vi "Read Sequential Addresses.vi"(7 "Target IC (1-8)":u8, 8 "error in (no error)":errorcluster, 9 "Addresses to Read":u16 format="%0.0f", 10 "Starting Address":u16 format="%04x", 11 "FPGA Interface in":refnum<class "FPGA Interface.lvclass">) -> (0 "error out":errorcluster, 2 "Data":u16[](array[numeric]) format="%04x")   [LabVIEW 2020, in "BCI-1553 API.lvlib" / "FPGA Interface.lvlib" / "FPGA Interface.lvclass"]
doc: "Reads a series of consecutive addresses from a component in the 1553 Session. Sequential addressing cannot be used on addresses from 0x0400 to 0x0800. This command blocks until it receives data back from the specified component."
uses:
  FPGA Interface.lvclass
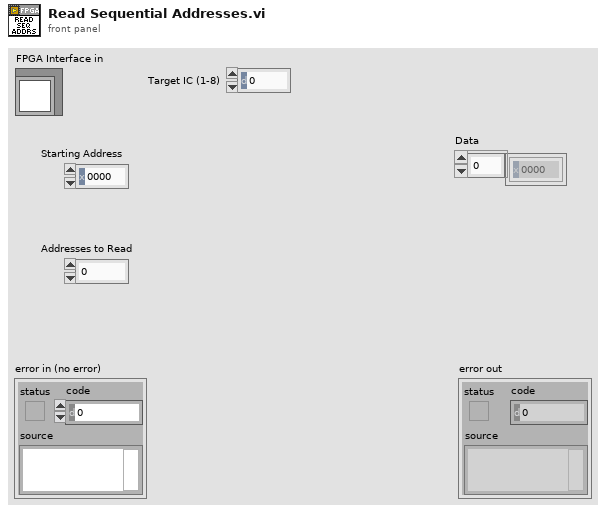
[diagram p1: front panel]
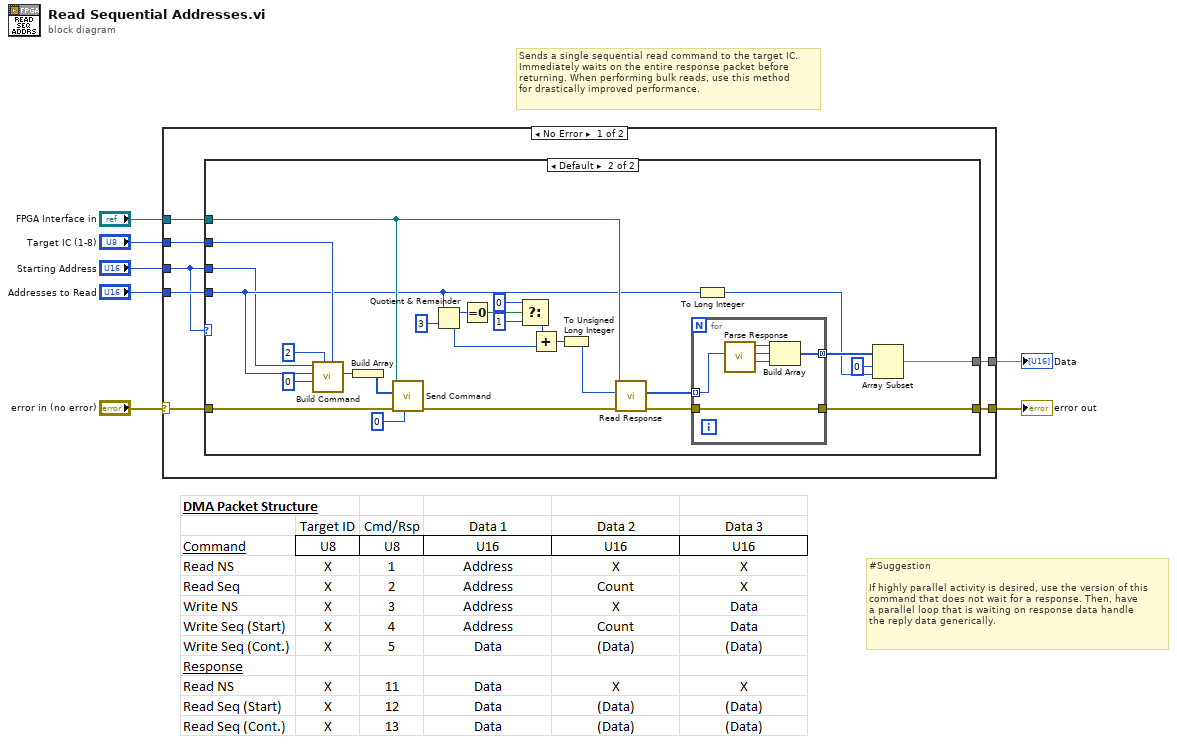
[diagram p0: block diagram]
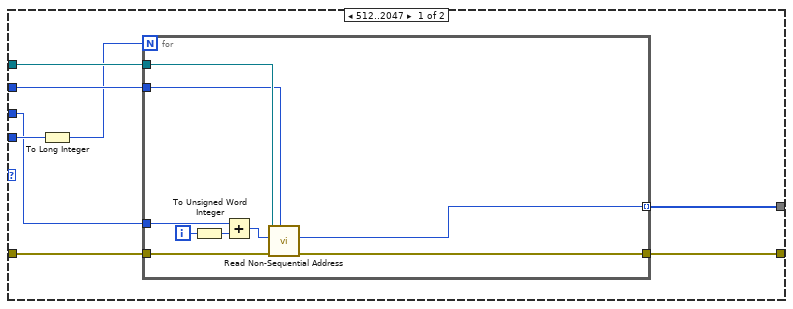
[diagram p2: hidden frame]
diagram:
  # "Sends a single sequential read command to the target IC.\nImmediately waits on the entire response packet before\nreturning. When performing bulk reads, use this method\nfor drastically improved performance."
  # "#Suggestion\n\nIf highly parallel activity is desired, use the version of this\ncommand that does not wait for a response. Then, have\na parallel loop that is waiting on response data handle\nthe reply data generically."
  n1 = case shown="No Error" "error in (no error)" {
    selector: "error in (no error)" -> [w14 w65]
    tunnel: [w11 w65] -> w6
    tunnel: "FPGA Interface in" -> [w12 _]
    tunnel: "Target IC (1-8)" -> [w13 _]
    tunnel: "Starting Address" -> [w8 _]
    tunnel: "Addresses to Read" -> [w9 _]
    tunnel: [w10 _] -> w1
    frame No Error {
      n2 = case shown="Default" w8 {
        tunnel: w14 -> [w17 w54]
        tunnel: w13 -> [w21 w53]
        tunnel: w12 -> [w22 w52]
        tunnel: [w16 w49] -> w11
        tunnel: [w15 w44] -> w10
        tunnel: w9 -> [w20 w43]
        tunnel: w8 -> [w18 w33]
        frame 512..2047 {
          n3 = To Long Integer(number=w20) -> (32bit integer=w19:i32)
          n4 = for {
            N: w19 -> [_]
            tunnel: w22 -> [w31]
            tunnel: w21 -> [w30]
            tunnel: w18 -> [w27]
            tunnel: w17 -> [w25]
            tunnel: [w24] -> w16
            tunnel: [w23] -> w15 mode=indexing
            i -> [w28]
            n5 = To Unsigned Word Integer(number=w28) -> (unsigned 16bit integer=w29:u16)
            n6 = Add(x=w27, y=w29) -> (x+y=w26:u16)
            n7 = call-dynamic "Read Non-Sequential Address.vi"("Target IC (1-8)"=w30, "error in (no error)"=w25, "Address"=w26, "FPGA Interface in"=w31) -> ("error out"=w24:errorcluster, "Data"=w23:u16)  [unwired: 6 in]
          }
        }
        frame Default {
          n8 = call "Build Command.vi"("Target"=w53, "CMD ID"=u8 2, "Data 3"=u16 0, "Data 2"=w43, "Data 1"=w33) -> ("Command"=w58:u64)  [unwired: 5 in, 1 out]
          n9 = Build Array(w58) -> (w57:u64[])
          n10 = call "Send Command.vi"("Timeout (ms)"=0, "error in (no error)"=w54, "Data"=w57, "FPGA Interface in"=w52) -> ("error out"=w56:errorcluster)  [unwired: 7 in]
          n11 = Quotient & Remainder(x=w43, y=u16 3) -> (x-y*floor(x/y)=w38:u16, floor(x/y)=w40:u16)
          n12 = Equal To 0?(x=w38) -> (x = 0?=w37:bool)
          n13 = Select(t=u16 0 ("y"), s=w37, f=u16 1 ("y")) -> (s? t:f=w36:u16)
          n14 = Add(x=w36, y=w40) -> (x+y=w39:u16)
          n15 = To Unsigned Long Integer(number=w39) -> (unsigned 32bit integer=w41:u32)
          n16 = call "Read Response.vi"("error in (no error)"=w56, "Number of Elements"=w41, "FPGA Interface in"=w52) -> ("error out"=w48:errorcluster, "Data"=w47:u64[])  [unwired: 6 in, 1 out]
          n17 = for {
            tunnel: [w64] -> w49
            tunnel: w48 -> [w64]
            tunnel: w47 -> [w63] mode=indexing
            tunnel: [w59] -> w46 mode=concatenating
            n18 = call "Parse Response.vi"("Data"=w63) -> ("Data 3"=w60:u16, "Data 2"=w61:u16, "Data 1"=w62:u16)  [unwired: 5 in, 3 out]
            n19 = Build Array(w62, w61, w60) -> (w59:u16[])
          }
          n20 = To Long Integer(number=w43) -> (32bit integer=w42:i32)
          n21 = Array Subset(array=w46, index=0, length=w42) -> (w44:u16[])
        }
      }
    }
    frame Error {
    }
  }
  "error out" <- w6
  "Data" <- w1
